vi "Measuring Complete - AndreTec-3.vi"() -> ()   [LabVIEW 2014]
doc: "André Romero - 2016\nandretec@ifsc.usp.br\nIFSC - USP"
uses:
  <vilib>/Analysis/Matrix/Datatypes/RealMatrix.ctl
  C:/Users/user/Documents/Andre/AutoLAB/Autolab SDK 1.11/EcoChemie.Autolab.Sdk.dll
  EcoChemie.Autolab.Sdk.dll
  <vilib>/Instr/_visa.llb/VISA Configure Serial Port (Instr).vi
  <vilib>/Utility/file.llb/Write To Spreadsheet File (DBL).vi
  <vilib>/Analysis/Matrix/NI_Matrix.lvlib
panel:
  in  "String":string
  in  "Start Measurement":bool
  out "Sensor":i32=1
  out "error out":errorcluster={"status"=TRUE, "code"=-1073807343, "source"="Property Node (arg 1) in VISA Configure Serial Port (Instr).vi->Measuring Complete - AndreTec-2.vi"}
  out "VISA resource name out":refnum<visa-resource-name>="COM3"
  in  "N. Sensors":i32=3 min=1 max=8
  out "Measured":cluster{dbl[], dbl[]}(graph)
  out "Points":i32=478
  in  "Abort":bool
  in  "Y axis Signal":string(combo)="WE(1).Current"
  in  "X axis Signal":string(combo)="WE(1).Potential"
  out "Measured data":cluster{"Y":dbl[], "Y":dbl[]}[](graph)
  out "X axis value":dbl=-1.1810302734375e-08
  out "Y axis value":dbl=3.0517578124972244e-06
  out "Measurement active":bool
  out "Blacklisted Commands detected":bool
  in  "Load Procedure":path=path "C:/Users/user/Documents/My Procedures 1.11/Procedures/bla.nox"
  out "Autolab Connected":bool
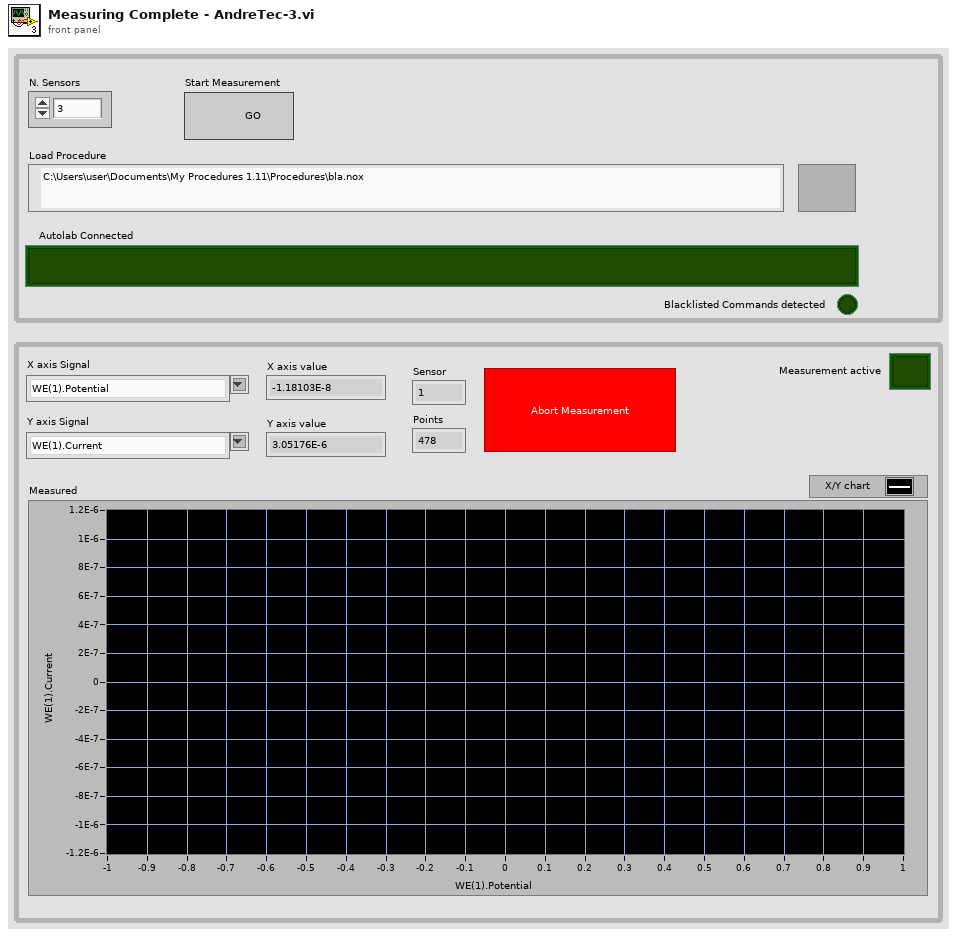
[diagram p1: front panel]
types:
  T1 = typedef "NI_Matrix.lvlib/RealMatrix.ctl" = dbl[][]
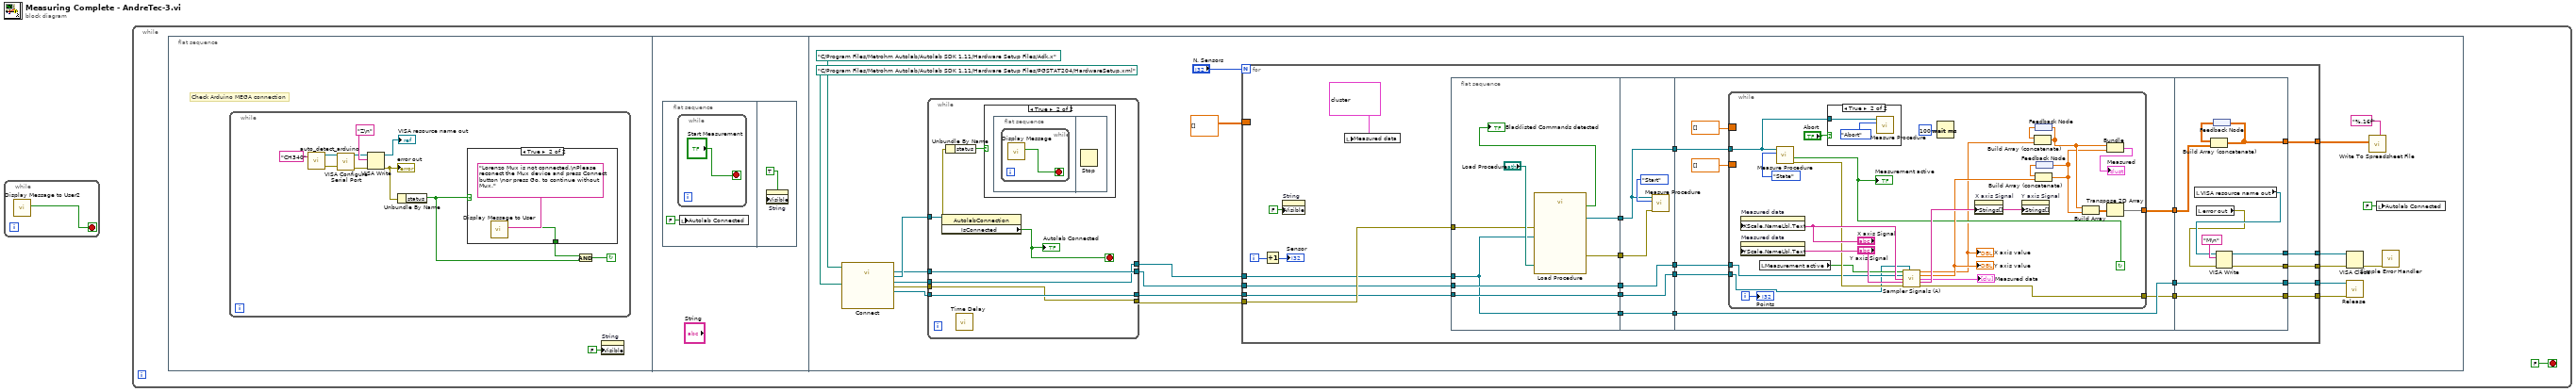
[diagram p0: block diagram]
diagram:
  n1 = while {
    stop <- w1 stop-if-true
    n2 = call "Display Message to User2"() -> ("OK"=w1:bool)  [unwired: 10 in, 1 out]
  }
  n3 = while {
    stop <- FALSE stop-if-true
    n4 = flat-sequence {
      frame #0 {
        # "Check Arduino MEGA connection"
        n5 = while {
          stop <- w6 continue-if-true
          n6 = call "auto_detect_arduino.vi"("instr name"="CH340") -> ("VISA resource name"=w14:refnum<visa-resource-name>, "error out"=w7:errorcluster)  [unwired: 1 in, 1 out]
          n7 = call-poly "VISA Configure Serial Port"("VISA resource name"=w14, "error in (no error)"=w7) -> ("VISA resource name out"=w11:refnum<visa-resource-name>, "error out"=w10:errorcluster)  [unwired: 7 in, 5 out]
          n8 = VISA Write(VISA resource name=w11, write buffer="Z\n" ("Command"), error in (no error)=w10) -> (VISA resource name out=→"VISA resource name out":refnum<visa-resource-name>, error out=w8:errorcluster)  [unwired: 1 out]
          "error out" <- w8
          n9 = Unbundle By Name(w8) -> ("status"=w5:bool)
          n10 = case shown="True" w5 {
            tunnel: [_ w15] -> w4
            frame False {
            }
            frame True {
              n11 = call "Display Message to User"("Message"="Lorenzo Mux is not connected.\nPlease reconect the Mux device and press Connect button \nor press Go, to continue without Mux.") -> ("Connect"=w15:bool)  [unwired: 9 in, 1 out]
            }
          }
          n12 = And(x=w4, y=w5) -> (x .and. y?=w6:bool)
        }
        n13 = property on="String" class="Str"("Visible"=FALSE) -> ()  [unwired: 2 in, 2 out]
      }
      frame #1 {
        n14 = flat-sequence {
          frame #0 {
            n15 = while {
              stop <- "Start Measurement" stop-if-true
            }
            n16 = local write "Autolab Connected"(FALSE ("Autolab Connected")) -> ()
          }
          frame #1 {
            n17 = property on="String" class="Str"("Visible"=TRUE) -> ()  [unwired: 2 in, 2 out]
          }
        }
      }
      frame #2 {
        n18 = call "Connect.vi"("Embedded Exe File"=path "C:/Program Files/Metrohm Autolab/Autolab SDK 1.11/Hardware Setup Files/Adk.x", "Hardware Setup File"=path "C:/Program Files/Metrohm Autolab/Autolab SDK 1.11/Hardware Setup Files/PGSTAT204/HardwareSetup.xml") -> ("Sampler"=w27:refnum<k24>, "AutolabConnection"=w32:refnum<k24>, "instrument"=w25:refnum<k24>, "Ei"=w20:refnum<k24>, "error out"=w22:errorcluster)  [unwired: 1 in, 8 out]
        n19 = while {
          tunnel: w32 -> [w47]
          tunnel: w27 -> [w44]
          tunnel: [w44] -> w26
          tunnel: w25 -> [w43]
          tunnel: [w43] -> w24
          tunnel: w20 -> [w42]
          tunnel: [w42] -> w23
          tunnel: w22 -> [w41]
          tunnel: [w41] -> w21
          stop <- w48 stop-if-true
          n20 = property class="AutolabConnection"(reference=w47) -> (error out=w45:errorcluster, "IsConnected"=w48:bool)  [unwired: 1 in, 1 out]
          "Autolab Connected" <- w48
          n21 = Unbundle By Name(w45) -> ("status"=w46:bool)
          n22 = call "Time Delay"() -> ()  [unwired: 2 in, 10 out]
          n23 = case shown="True" w46 {
            frame False {
            }
            frame True {
              n24 = flat-sequence {
                frame #0 {
                  n25 = while {
                    stop <- w49 stop-if-true
                    n26 = call "Display Message"() -> ("OK"=w49:bool)  [unwired: 10 in, 1 out]
                  }
                }
                frame #1 {
                  n27 = Stop() -> ()  [unwired: 1 in]
                }
              }
            }
          }
        }
        n28 = for {
          N: "N. Sensors" -> [_]
          tunnel: [w63] -> w40
          tunnel: [w62] -> w39
          tunnel: [w61] -> w36
          tunnel: [w60] -> w35
          tunnel: w21 -> [w59]
          tunnel: w24 -> [w58]
          tunnel: w26 -> [w57]
          tunnel: w23 -> [w56]
          tunnel: [w53] -> w31
          border: T1 [] ("Real Matrix") -> [_]
          i -> [w52]
          n29 = Increment(x=w52) -> (x+1=→"Sensor":i32)
          n30 = property on="String" class="Str"("Visible"=FALSE) -> ()  [unwired: 2 in, 2 out]
          n31 = local write "Measured data"(cluster{"Y":dbl[], "Y":dbl[]}[] [{"Y"=array[2393 elements], "Y"=array[2393 elements]}] ("Measured data")) -> ()
          n32 = flat-sequence {
            tunnel: [w80] -> w74
            tunnel: [w79] -> w73
            tunnel: [w77] -> w72
            tunnel: [w76] -> w71
            tunnel: [w75] -> w70
            tunnel: w58 -> [w75]
            tunnel: w59 -> [w78]
            tunnel: w57 -> [w77]
            tunnel: w56 -> [w76]
            tunnel: w74 -> [w86]
            tunnel: w73 -> [w87]
            tunnel: [w86] -> w69
            tunnel: w72 -> [w85]
            tunnel: w71 -> [w84]
            tunnel: [w85] -> w68
            tunnel: [w84] -> w67
            tunnel: [w83] -> w66
            tunnel: w70 -> [w83]
            tunnel: w69 -> [w96]
            tunnel: w68 -> [w95]
            tunnel: w67 -> [w94]
            tunnel: w66 -> [w93]
            tunnel: [w93] -> w65
            tunnel: [w89] -> w64
            tunnel: [w92] -> w54
            tunnel: w65 -> [w132]
            tunnel: w64 -> [w131]
            tunnel: [w132] -> w63
            tunnel: [w131] -> w62
            tunnel: [w127] -> w61
            tunnel: [w126] -> w60
            tunnel: w54 -> [w125]
            tunnel: [w123] -> w53
            frame #0 {
              n33 = call "Load Procedure.vi"("error in (no error)"=w78, "Procedure"="Load Procedure", "Instrument"=w75) -> ("error out"=w79:errorcluster, "Contains"=→"Blacklisted Commands detected":bool, "LoadProcedure"=w80:refnum<k24>)  [unwired: 6 out]
            }
            frame #1 {
              n34 = call "Measure Procedure.vi"("error in"=w87, "Request for procedure"=enum16{"State", "Save", "Abort", "Start"}."Start", "LoadProcedure"=w86) -> ()  [unwired: 1 in, 8 out]
            }
            frame #2 {
              n35 = while {
                tunnel: w96 -> [w112]
                tunnel: w95 -> [w113]
                tunnel: w94 -> [w97]
                tunnel: [w100] -> w92
                border: dbl[] [] -> [_]
                border: dbl[] [] -> [_]
                tunnel: [w99] -> w89
                i -> [w109]
                stop <- w104 continue-if-true
                n36 = property on="Measured data" class="XYGraph (strict)"("XScale.NameLbl.Text"="X axis Signal") -> ()  [unwired: 2 in, 2 out]
                n37 = property on="Measured data" class="XYGraph (strict)"("YScale.NameLbl.Text"="Y axis Signal") -> ()  [unwired: 2 in, 2 out]
                n38 = local read "Measurement active"() -> (w115:bool)
                n39 = call "Measure Procedure.vi"("Request for procedure"=enum16{"State", "Save", "Abort", "Start"}."State", "LoadProcedure"=w112) -> ("error out"=w116:errorcluster, "IsMeasuring"=w104:bool)  [unwired: 2 in, 6 out]
                "Measurement active" <- w104
                n40 = case shown="True" "Abort" {
                  tunnel: w112 -> [_ w121]
                  frame False {
                  }
                  frame True {
                    n41 = call "Measure Procedure.vi"("Request for procedure"=enum16{"State", "Save", "Abort", "Start"}."Abort", "LoadProcedure"=w121) -> ()  [unwired: 2 in, 8 out]
                  }
                }
                n42 = call "Sampler Signals (A).vi"("IsMeasuring"=w115, "EI"=w97, "Sampler"=w113, "Signal X"="X axis Signal", "Signal Y"="Y axis Signal", "error in"=w116) -> ("X"=w98:dbl, "Y"=w106:dbl, "XY Graph"=→"Measured data":cluster{"Y":dbl[], "Y":dbl[]}[], "GetSignals"=w118:string[], "error out"=w99:errorcluster)  [unwired: 4 in, 1 out]
                "Y axis value" <- w106
                "X axis value" <- w98
                n43 = Wait (ms)(milliseconds to wait=u32 100) -> ()  [unwired: 1 out]
                n44 = property on="X axis Signal" class="CmbBox"("Strings[]"=w118) -> ()  [unwired: 2 in, 2 out]
                n45 = property on="Y axis Signal" class="CmbBox"("Strings[]"=w118) -> ()  [unwired: 2 in, 2 out]
                n46 = feedback #1() -> (w108:dbl[])
                n47 = Build Array (concatenate)(w108, w98) -> (w102:dbl[])
                n48 = feedback-in #1(w102) -> ()
                n49 = feedback #2() -> (w107:dbl[])
                n50 = Build Array (concatenate)(w107, w106) -> (w101:dbl[])
                n51 = feedback-in #2(w101) -> ()
                n52 = Build Array(w102, w101) -> (w103:dbl[][])
                n53 = Bundle(w102, w101) -> (→"Measured":cluster{dbl[], dbl[]})  [unwired: 1 in]
                n54 = Transpose 2D Array(2D array=w103) -> (transposed array=w100:dbl[][])
                "Points" <- w109
              }
            }
            frame #3 {
              n55 = local read "VISA resource name out"() -> (w129:refnum<visa-resource-name>)
              n56 = local read "error out"() -> (w128:errorcluster)
              n57 = feedback #3() -> (w124:T1)
              n58 = Build Array (concatenate)(w124, w125) -> (w123:T1)
              n59 = feedback-in #3(w123) -> ()
              n60 = VISA Write(VISA resource name=w129, write buffer="M\n" ("Command"), error in (no error)=w128) -> (VISA resource name out=w127:refnum<visa-resource-name>, error out=w126:errorcluster)  [unwired: 1 out]
            }
          }
        }
        n61 = call "Release.vi"("error in (no error)"=w39, "Instrument"=w40) -> ()  [unwired: 1 in, 9 out]
        n62 = VISA Close(VISA resource name=w36, error in (no error)=w35) -> (error out=w37:errorcluster)
        n63 = call-poly <vilib>:"Write To Spreadsheet File.vi"("format (%.3f)"="%.16f", "2D data"=w31) -> ()  [unwired: 6 in, 1 out]
        n64 = local write "Autolab Connected"(FALSE ("Autolab Connected")) -> ()
        n65 = call <vilib>:"Simple Error Handler.vi"("error in (no error)"=w37) -> ()  [unwired: 1 in, 8 out]
      }
    }
  }
